vi "NISE.Commit Properties for Devices.vi"(0 "SLSC Interface in":refnum<class "SLSC Interface.lvclass">, 5 "devices":refnum<k21>="$DefaultDevices", 11 "error in (no error)":errorcluster) -> (4 "SLSC Interface out":refnum<class "SLSC Interface.lvclass">, 15 "error out":errorcluster)   [LabVIEW 2016, in "SLSC Interface.lvclass"]
uses:
  SLSC Interface.lvclass
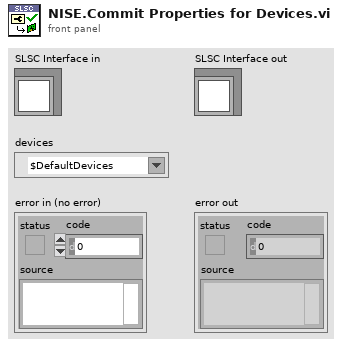
[diagram p1: front panel]
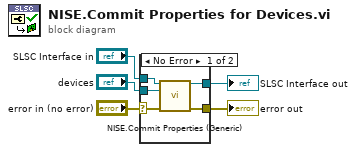
[diagram p0: block diagram]
diagram:
  n1 = case shown="No Error" "error in (no error)" {
    selector: "error in (no error)" -> [w7 w12]
    tunnel: [w6 w12] -> w4
    tunnel: [w9 w11] -> w2
    tunnel: "SLSC Interface in" -> [w10 w11]
    tunnel: "devices" -> [w8 _]
    frame No Error {
      n2 = call "NISE.Commit Properties (Generic).vi"("SLSC Interface in"=w10, "resources"=w8, "error in (no error)"=w7) -> ("SLSC Interface out"=w9:refnum<class "SLSC Interface.lvclass">, "error out"=w6:errorcluster)  [unwired: 11 in]
    }
    frame Error {
    }
  }
  "error out" <- w4
  "SLSC Interface out" <- w2
